vi "Meal Calculator.vi"() -> ()   [LabVIEW 2010]
doc: "A sample VI demonstrating how to use value types and coercion to solve a simple mathematical application."
panel:
  in  "Side":enum16{"Onion Rings", "Salad"}(ring)
  in  "Drink":enum16{"Water", "Juice"}(ring)
  in  "Tax Percentage":dbl
  out "Total Price":dbl format="%#.2g"
  in  "# of Sides":i32
  in  "# of Drinks":i32
  in  "# of Mains":i32
  in  "Main":enum16{"Chicken Nuggets", "Chicken Sandwich"}(ring)
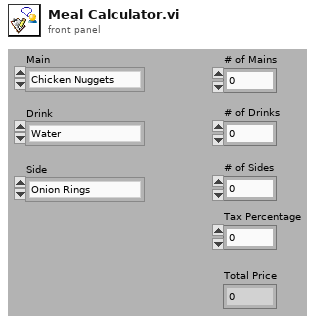
[diagram p1: front panel]
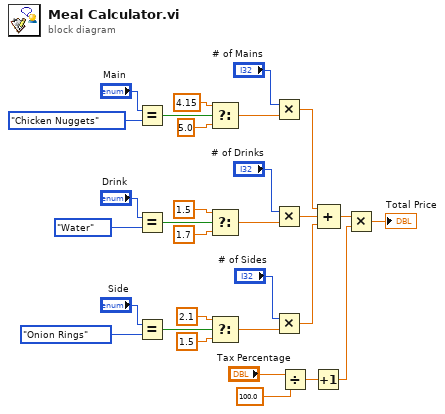
[diagram p0: block diagram]
diagram:
  n1 = Equal?(x="Main", y=enum16{"Chicken Nuggets", "Chicken Sandwich"}."Chicken Nuggets") -> (x = y?=w22:bool)
  n2 = Equal?(x="Drink", y=enum16{"Water", "Juice"}."Water" ("Drink")) -> (x = y?=w16:bool)
  n3 = Equal?(x="Side", y=enum16{"Onion Rings", "Salad"}."Onion Rings" ("Side")) -> (x = y?=w12:bool)
  n4 = Select(t=4.15, s=w22, f=5.0) -> (s? t:f=w19:dbl)
  n5 = Select(t=1.5, s=w16, f=1.7) -> (s? t:f=w14:dbl)
  n6 = Select(t=2.1, s=w12, f=1.5) -> (s? t:f=w9:dbl)
  n7 = Multiply(x="# of Mains", y=w19) -> (x*y=w29:dbl)
  n8 = Multiply(x="# of Drinks", y=w14) -> (x*y=w28:dbl)
  n9 = Multiply(x="# of Sides", y=w9) -> (x*y=w27:dbl)
  n10 = Divide(x="Tax Percentage", y=100.0) -> (x/y=w4:dbl)
  n11 = Increment(x=w4) -> (x+1=w24:dbl)
  n12 = Compound Arithmetic op=ADD(w29, w28, w27) -> (w26:dbl)
  n13 = Multiply(x=w26, y=w24) -> (x*y=→"Total Price":dbl)
